vi "Render String Partial.vi"(8 "Error In":errorcluster) -> (0 "Error Out":errorcluster)   [LabVIEW 2018, in "Tests.lvlib" / "Render.lvlib"]
uses:
  Render.lvlib
  <vilib>/addons/_JKI Toolkits/Caraya/classes/Test/Test.lvclass
  <vilib>/addons/_JKI Toolkits/Caraya/classes/Assert/Assert.lvclass
  src/Toolkit/Toolkit.lvlib
  src/Toolkit/Data/Map/Map.lvclass
  src/Toolkit/Low-Level/Loaders/String/String.lvclass
  src/Toolkit/Low-Level/Support/Render to String.vi
  src/Toolkit/Low-Level/Support/Lex String.vi
  src/Toolkit/Data/Map/Support/From String.vi
  src/Toolkit/Low-Level/Context/Compiler.lvclass
  D:/Users/cfield/Code/Field R&D Services/Labstache/src/Toolkit/Low-Level/Loaders/Loader/Loader.lvclass
  D:/Users/cfield/Code/Field R&D Services/Labstache/src/Toolkit/Data/Datum/Datum.lvclass
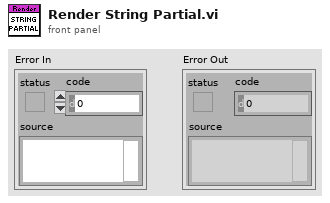
[diagram p1: front panel]
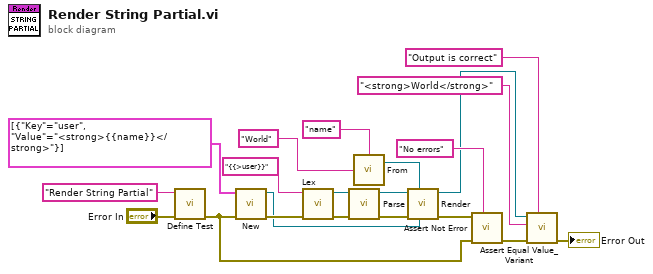
[diagram p0: block diagram]
diagram:
  n1 = call <vilib>:"Define Test.vi"("error in (no error)"="Error In", "Label (VI Title)"="Render String Partial") -> ("error out"=w4:errorcluster)  [unwired: 9 in]
  n2 = call "New.vi"("Error In"=w4, "Key-Value Pairs"=cluster{"Key":string, "Value":string}[] [{"Key"="user", "Value"="<strong>{{name}}</strong>"}]) -> ("Error Out"=w8:errorcluster, "String"=w1:refnum<class "String.lvclass">)  [unwired: 8 in]
  n3 = call-poly "Lex.vi"("Error In"=w8, "Context In"="{{>user}}" ("format string")) -> ("Error Out"=w11:errorcluster, "Context Out"=w12:refnum<class "Compiler.lvclass">)  [unwired: 7 in, 1 out]
  n4 = call "Parse.vi"("Error In"=w11, "Context In"=w12) -> ("Error Out"=w13:errorcluster, "Context Out"=w9:refnum<class "Compiler.lvclass">)  [unwired: 7 in, 1 out]
  n5 = call-poly "From.vi"("Value"="World", "Key"="name") -> ("Map"=w10:refnum<class "Map.lvclass">)
  n6 = call-poly "Render.vi"("Loader"=w1, 7:w10, "Error In"=w13, "Context In"=w9) -> ("Error Out"=w15:errorcluster, "Context Out"=w14:refnum<class "Compiler.lvclass">)  [unwired: 5 in, 1 out]
  n7 = call <vilib>:"Assert Not Error.vi"("Label"="No errors", "error in (no error)"=w4, "Not Error?"=w15) -> ("error out"=w18:errorcluster)  [unwired: 8 in]
  n8 = call <vilib>:"Assert Equal Value_Variant.vi"("Label"="Output is correct", "error in (no error)"=w18, "Y"="<strong>World</strong>", "X"=w14) -> ("error out"=→"Error Out":errorcluster)  [unwired: 7 in]
